vi "CD Init.vi"(0 "Device Reference":T14 format="%.0x", 11 "Error (in)":errorcluster) -> (1 "Card Parameters (out)":T13, 3 "Output Channel Data []":T4[](array[typedef]) {"Labels Settings"."Word"."Param Setting"."Num Bits" min=1 max=32; "Labels Settings"."Word"."Param Setting"."Start Bit" min=8 max=31; "Labels Settings"."Label" format="%.0o"}, 4 "# of Output Channels":i32, 6 "# of Input Channels":i32, 10 "Refs":i32[](array[numeric]), 12 "Map":T3[](array[typedef]), 13 "Raw Values":T1, 14 "Input Channel Data []":T4[](array[typedef]) {"Labels Settings"."Word"."Param Setting"."Num Bits" min=1 max=32; "Labels Settings"."Word"."Param Setting"."Start Bit" min=8 max=31; "Labels Settings"."Label" format="%.0o"}, 15 "Error (out)":errorcluster)   [LabVIEW 2016, in "Ballard Arinc-429 Engine.lvlib"]
uses:
  Ballard Arinc-429 Engine.lvlib
  <vilib>/NI Veristand/Custom Device API/Custom Device Item Ref.ctl
  RT Controls/Card Parameters.ctl
  RT Controls/RT HW Channel.ctl
  RT Controls/RT Label Settings.ctl
  Shared/Controls and Global/Label.ctl
  Shared/Controls and Global/transferPeriod.ctl
  RT Controls/RT Word Settings.ctl
  RT Controls/RT Param Setting.ctl
  Shared/Controls and Global/Start Bit.ctl
  Shared/Controls and Global/Number of Bits.ctl
  Shared/Controls and Global/TransferType.ctl
  RT Controls/RT Tx Association.ctl
  RT Controls/RT Tx Default Raw Value.ctl
  RT Controls/RT Tx Default Raw Value_Association.ctl
  RT Controls/RT Init States.ctl
  <vilib>/NI Veristand/Custom Device API/Custom Device Channel Type.ctl
  <vilib>/NI Veristand/Custom Device Tools/Custom Device Utility Library/RT Debug String Color Spec.ctl
  Shared/Controls and Global/Global.vi
  <vilib>/NI Veristand/Custom Device API/Get Item Property (I32).vi
  <vilib>/NI Veristand/Custom Device API/Get Item Property (Variant).vi
  <vilib>/NI Veristand/Custom Device Tools/Custom Device Utility Library/NI VeriStand - Search for Item by GUID.vi
  <vilib>/NI Veristand/Custom Device API/Custom Device API.lvlib
  Shared/Ballard Arinc-429 Shared.lvlib
  <vilib>/NI Veristand/Custom Device Tools/Custom Device Utility Library/Custom Device Utility Library.lvlib
  <instrlib>/BTI429Lib/BTI429LV.lvlib
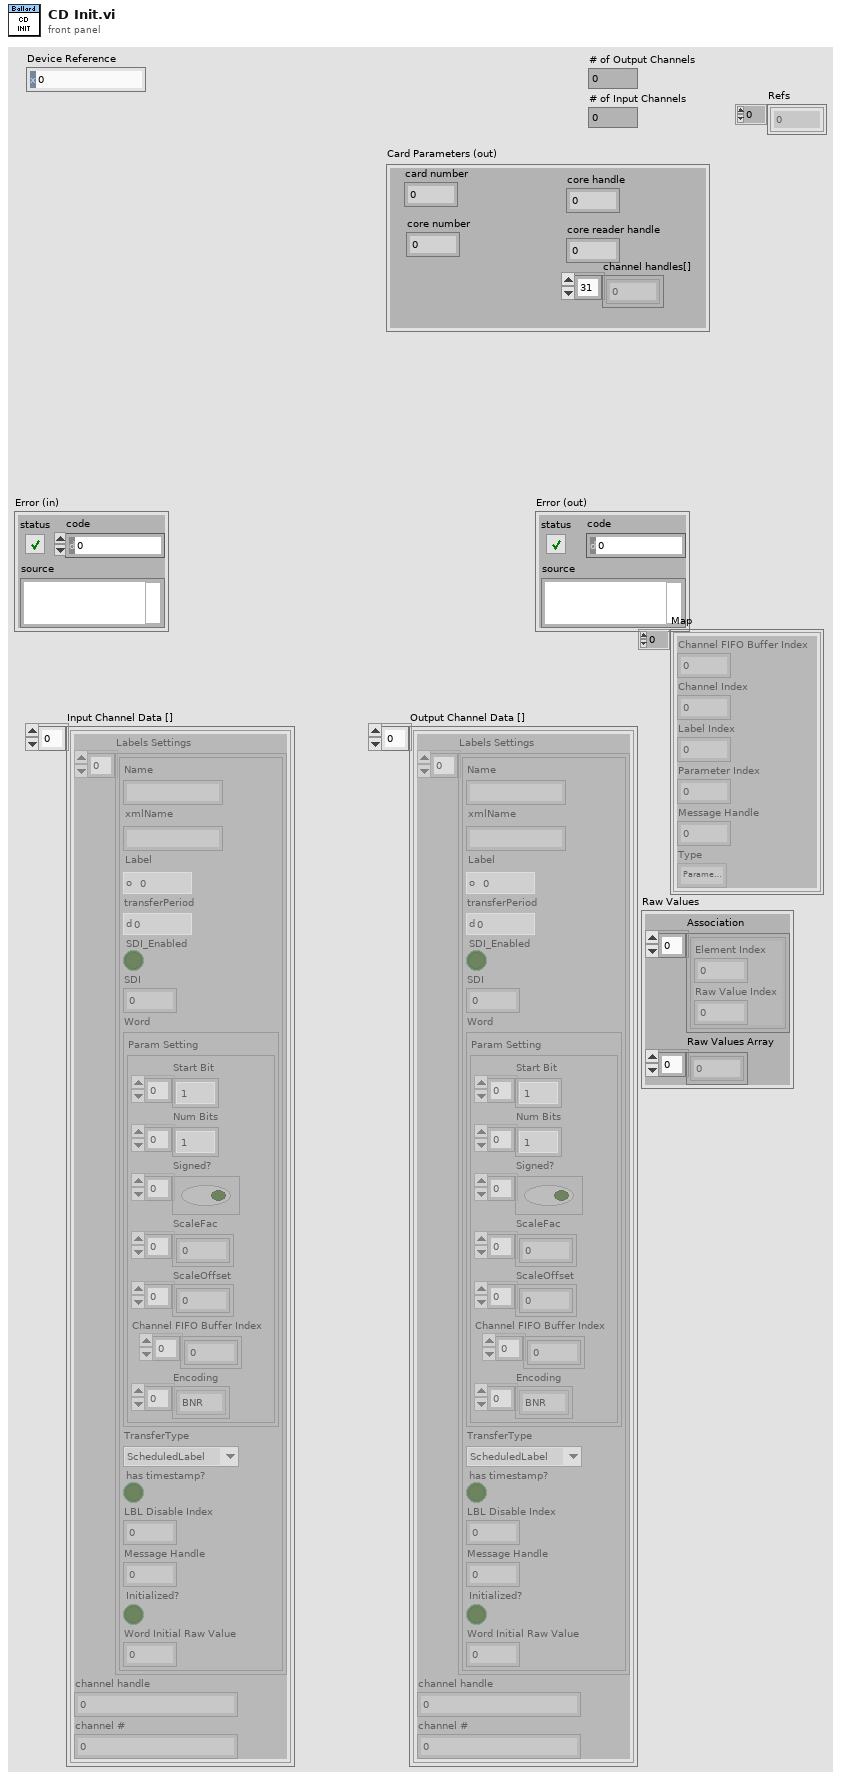
[diagram p1: front panel]
types:
  T1 = typedef "Ballard Arinc-429 Engine.lvlib/RT Tx Default Raw Value.ctl" = cluster{"Association":T2[], "Raw Values Array":u32[]}
  T2 = typedef "Ballard Arinc-429 Engine.lvlib/RT Tx Default Raw Value_Association.ctl" = cluster{"Element Index":i32, "Raw Value Index":i32}
  T3 = typedef "Ballard Arinc-429 Engine.lvlib/RT Tx Association.ctl" = cluster{"Channel FIFO Buffer Index":i32, "Channel Index":i32, "Label Index":i32, "Parameter Index":i32, "Message Handle":u64, "Type":enum16{"Parameter Channel", "Disable Channel"}}
  T4 = typedef "Ballard Arinc-429 Engine.lvlib/RT HW Channel.ctl" = cluster{"Labels Settings":T5[], "channel handle":u32, "channel #":u16}
  T5 = typedef "Ballard Arinc-429 Engine.lvlib/RT Label Settings.ctl" = cluster{"Name":string, "xmlName":string, "Label":T6, "transferPeriod":T7, "SDI_Enabled":bool, "SDI":u8, "Word":T8, "TransferType":T12, "has timestamp?":bool, "LBL Disable Index":i32, "Message Handle":u64, "Initialized?":bool, "Word Initial Raw Value":u32}
  T6 = typedef "Ballard Arinc-429 Shared.lvlib/Label.ctl" = u8
  T7 = typedef "Ballard Arinc-429 Shared.lvlib/transferPeriod.ctl" = u32
  T8 = typedef "Ballard Arinc-429 Engine.lvlib/RT Word Settings.ctl" = cluster{"Param Setting":T9}
  T9 = typedef "Ballard Arinc-429 Engine.lvlib/RT Param Setting.ctl" = cluster{"Start Bit":T10[], "Num Bits":T11[], "Signed?":bool[], "ScaleFac":dbl[], "ScaleOffset":dbl[], "Channel FIFO Buffer Index":i32[], "Encoding":enum16{"BNR", "BCD", "Discrete"}[]}
  T10 = typedef "Ballard Arinc-429 Shared.lvlib/Start Bit.ctl" = i32
  T11 = typedef "Ballard Arinc-429 Shared.lvlib/Number of Bits.ctl" = i32
  T12 = typedef "Ballard Arinc-429 Shared.lvlib/TransferType.ctl" = enum16{"ScheduledLabel", "Acyclic", "Block", "Strobe"}
  T13 = typedef "Ballard Arinc-429 Engine.lvlib/Card Parameters.ctl" = cluster{"card number":i32, "core number":i32, "core handle":u64, "core reader handle":u64, "channel handles[]":u64[]}
  T14 = typedef "Custom Device API.lvlib/Custom Device Item Ref.ctl" = u64
  T15 = typedef "Ballard Arinc-429 Engine.lvlib/RT Init States.ctl" = enum16{"Initialization", "Get Card Settings", "Get Channel Count", "Parse Channels", "Ballard-429 Initialize", "Get Status Channels Reference", "Exit"}
  T16 = typedef "Custom Device API.lvlib/Custom Device Channel Type.ctl" = enum16{"Input", "Output"}
  T17 = enum16{"open", "replace", "create", "open or create", "replace or create", "replace or create with confirmation"}
  T18 = typedef "Custom Device Utility Library.lvlib/RT Debug String Color Spec.ctl" = u16
  T19 = typedef "Custom Device API.lvlib/Custom Device File Dependency.ctl" = cluster{"Source":T20, "RT Destination":path, "ForceDownload?":bool, "SupportedTarget":T22, "Version":string}
  T20 = typedef "Custom Device API.lvlib/Path Specification.ctl" = cluster{"Path":path, "Type":T21}
  T21 = typedef "Custom Device API.lvlib/Path Type.ctl" = enum16{"Absolute", "To Base", "To Common Data Dir", "To Application Data Dir"}
  T22 = typedef "Custom Device API.lvlib/Custom Device Supported Target.ctl" = enum16{"All", "PharLap", "VxWorks", "Windows", "Linux_32_ARM", "Linux_x64", "PharLap & Windows", "PharLap & VxWorks", "VxWorks & Windows"}
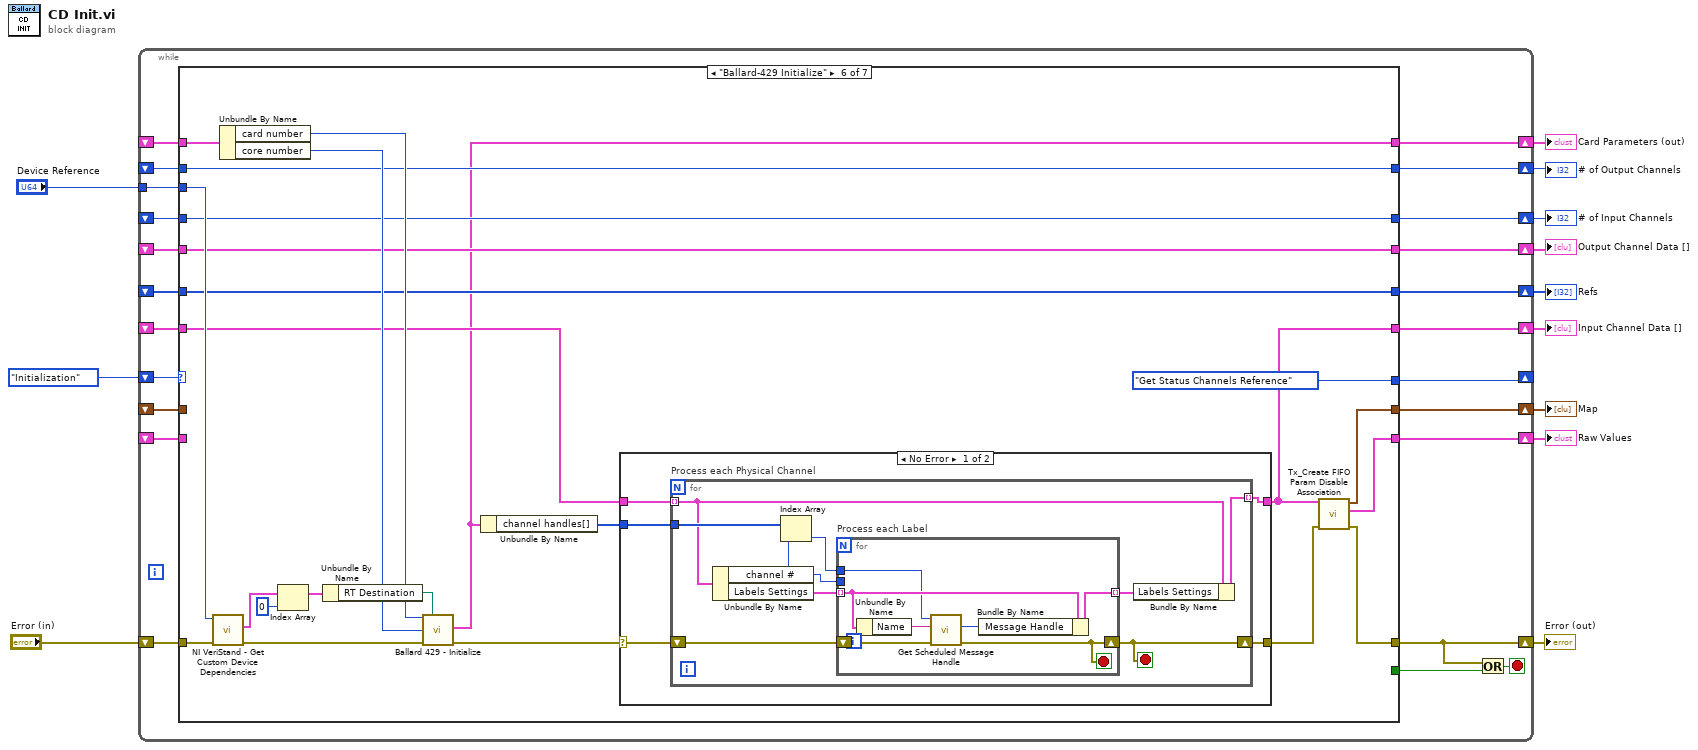
[diagram p0: block diagram]
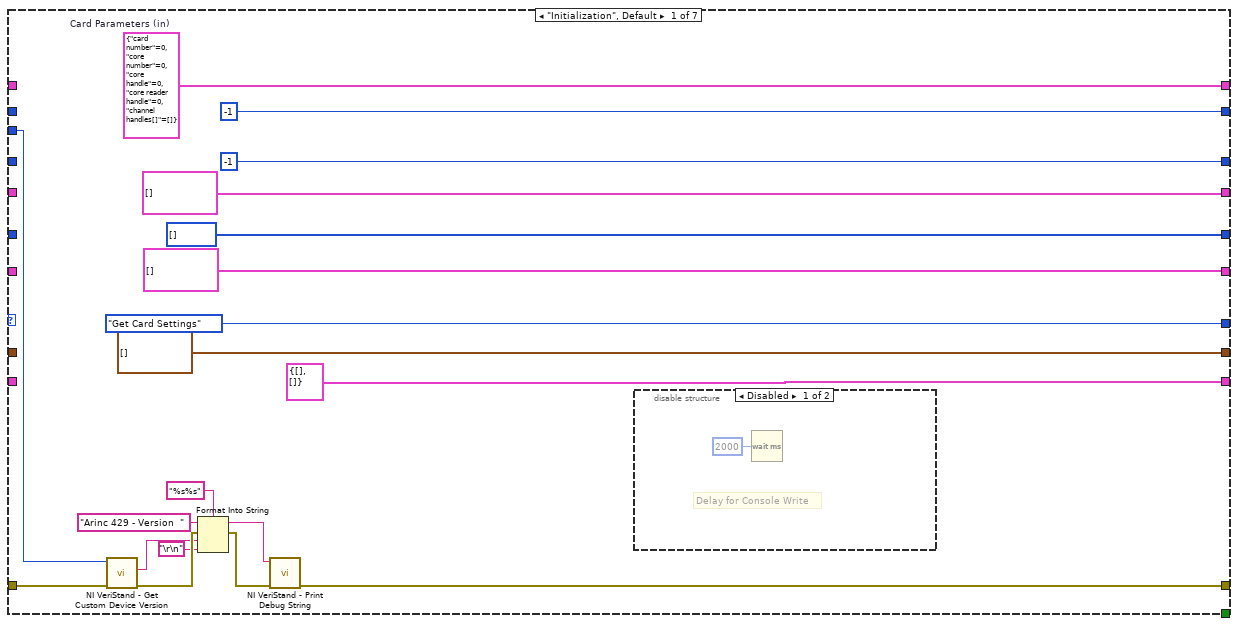
[diagram p2: hidden frame]
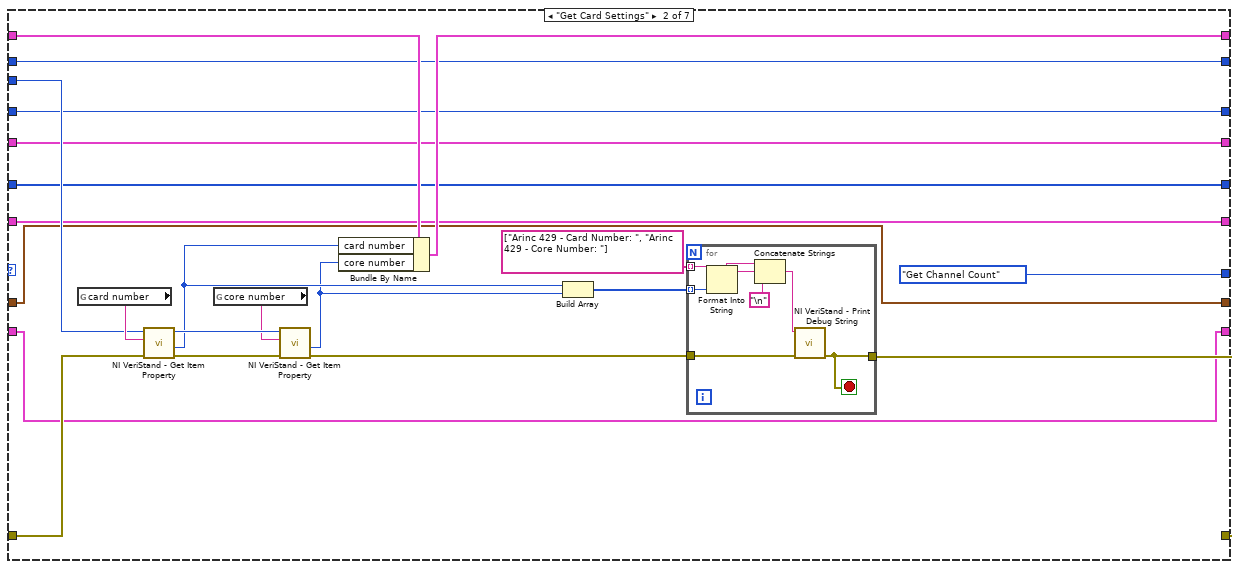
[diagram p4: hidden frame]
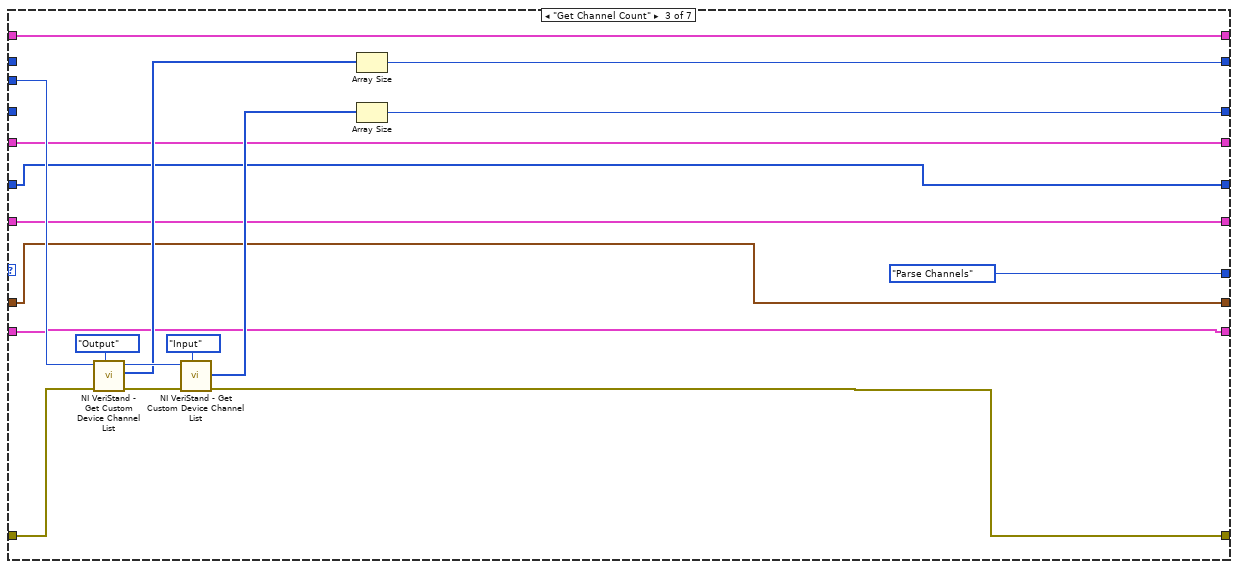
[diagram p5: hidden frame]
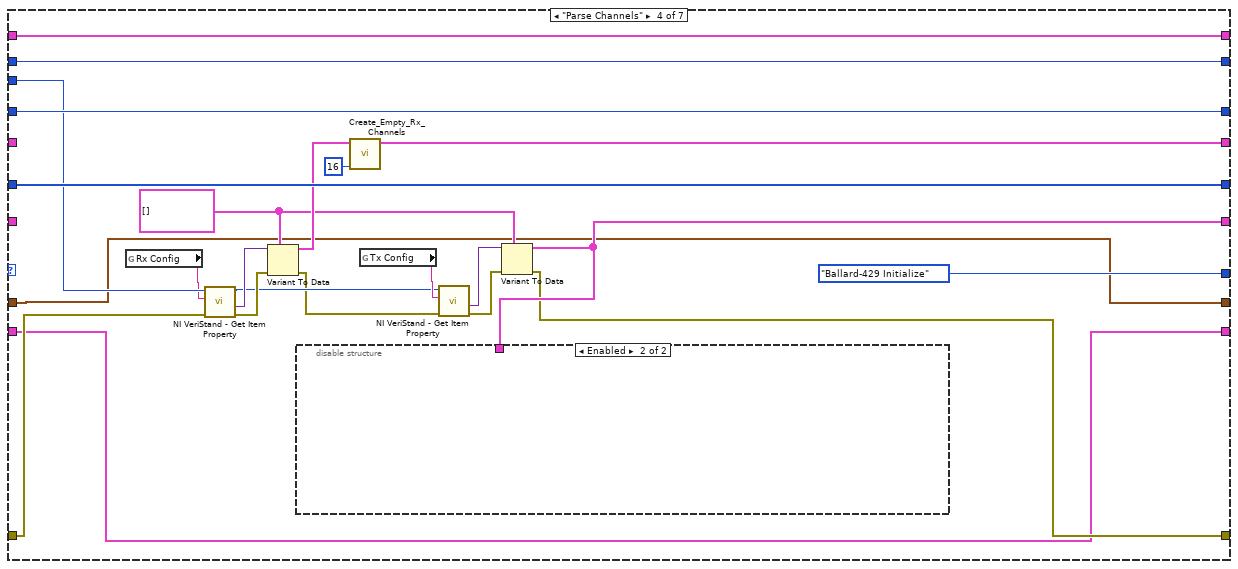
[diagram p6: hidden frame]
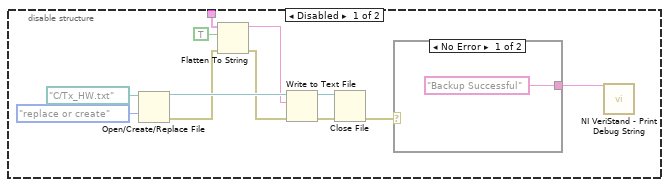
[diagram p7: hidden frame]
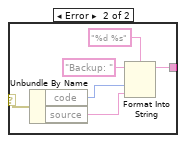
[diagram p8: hidden frame]
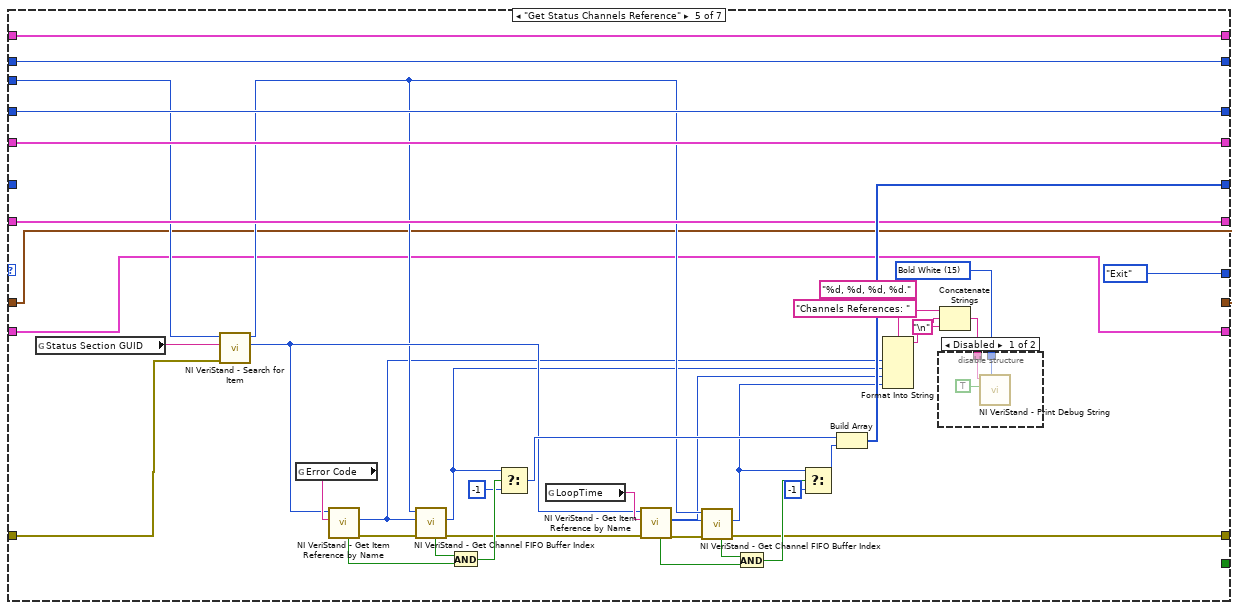
[diagram p9: hidden frame]
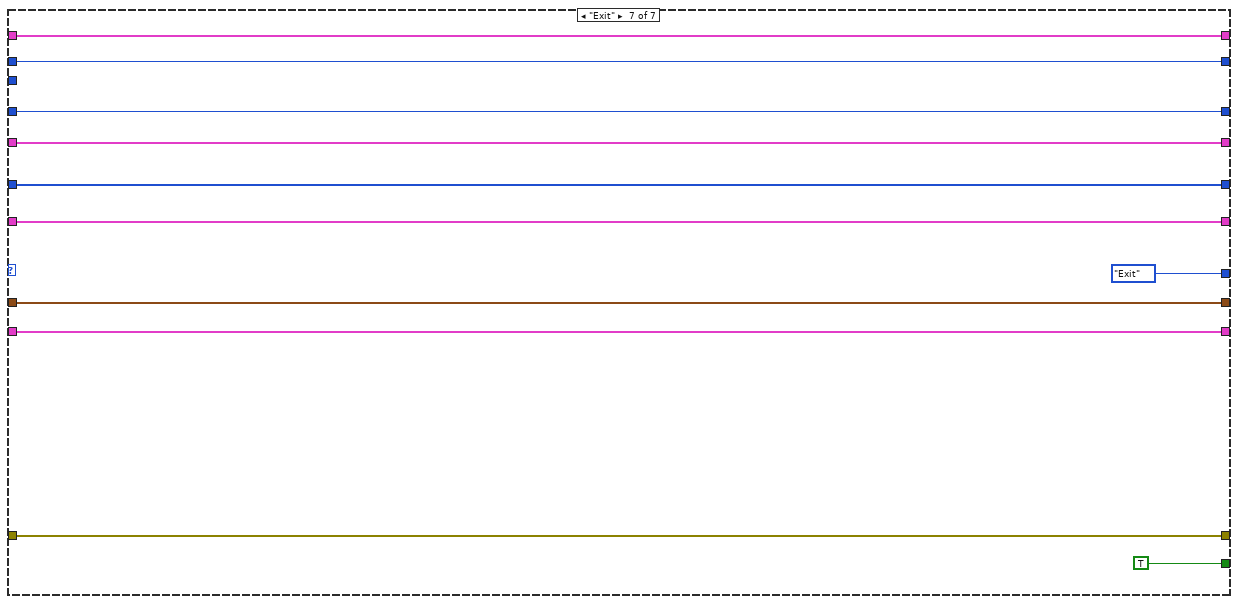
[diagram p12: hidden frame]
diagram:
  n1 = while {
    shift-right: [w34] -> _
    shift-left: RT_Init_States."Initialization" -> [w28]
    tunnel: "Device Reference" -> [w33]
    shift-right: [w29] -> w8
    shift-left: _ -> [w30]
    shift-right: [w27] -> w7
    shift-left: _ -> [w25]
    shift-right: [w26] -> w6
    shift-left: _ -> [w24]
    shift-right: [w23] -> w5
    shift-left: _ -> [w20]
    shift-right: [w22] -> w4
    shift-left: _ -> [w21]
    shift-right: [w19] -> w3
    shift-left: _ -> [w18]
    shift-right: [w17] -> w10
    shift-left: "Error (in)" -> [w35]
    shift-right: [w16] -> w2
    shift-left: _ -> [w15]
    shift-right: [w14] -> w1
    shift-left: _ -> [w13]
    stop <- w32 stop-if-true
    n2 = case shown="\"Ballard-429 Initialize\"" w28 {
      tunnel: w35 -> [w47 w72 w98 w106 w161 w204 w245]
      tunnel: [w45 w69 w85 w105 w162 w188 w245] -> w17
      tunnel: [RT_Init_States."Get Card Settings" RT_Init_States."Get Channel Count" RT_Init_States."Parse Channels" RT_Init_States."Ballard-429 Initialize" RT_Init_States."Exit" RT_Init_States."Get Status Channels Reference" RT_Init_States."Exit"] -> w34
      tunnel: w33 -> [w46 w67 w97 w118 w159 w203 _]
      tunnel: [_ _ _ _ _ _ TRUE] -> w31
      tunnel: w30 -> [_ w66 w93 w124 w174 w208 w242]
      tunnel: [w53 w65 w93 w124 w174 w196 w242] -> w29
      tunnel: [T4[] [] ("Rx Channels Out") w62 w91 w122 w184 w200 w239] -> w27
      tunnel: [T4[] [] ("Channel Data []") w61 w90 w107 w177 w192 w238] -> w26
      tunnel: w25 -> [_ w62 w91 _ w184 w200 w239]
      tunnel: w24 -> [_ w61 w90 _ w177 w201 w238]
      tunnel: [-1 w59 w92 w120 w183 w199 w240] -> w23
      tunnel: [-1 w60 w88 w121 w182 w198 w241] -> w22
      tunnel: w21 -> [_ w60 _ w121 w182 w198 w241]
      tunnel: w20 -> [_ w59 _ w120 w183 w199 w240]
      tunnel: [i32[] [] w58 w89 w119 w178 w197 w237] -> w19
      tunnel: w18 -> [_ w58 w89 w119 _ w197 w237]
      tunnel: [T3[] [] ("Map") w57 w87 w104 w146 w190 w236] -> w16
      tunnel: w15 -> [_ w57 w87 w104 w146 _ w236]
      tunnel: [T1 {"Association"=[], "Raw Values Array"=[]} ("Raw Values") w56 w86 w103 w145 w189 w235] -> w14
      tunnel: w13 -> [_ w56 w86 w103 w145 _ w235]
      frame "Initialization", Default {
        w53 = T13 {"card number"=0, "core number"=0, "core handle"=0, "core reader handle"=0, "channel handles[]"=[]}  # Card Parameters (in)
        n3 = call <vilib>:"NI VeriStand - Get Custom Device Version.vi"("error in (no error)"=w47, "Device Ref in"=w46) -> ("error out"=w44:errorcluster, "Value"=w41:string)  [unwired: 7 in, 1 out]
        n4 = Format Into String(format string="%s%s", initial string="Arinc 429 - Version  ", error in=w44, w41, "\r\n") -> (resulting string=w39:string, error out=w43:errorcluster)
        n5 = call <vilib>:"NI VeriStand - Print Debug String.vi"("error in (no error)"=w43, "Message"=w39) -> ("error out"=w45:errorcluster)  [unwired: 9 in]
        n6 = disable-structure shown="Disabled" {
          frame Disabled {
            # "Delay for Console Write"
            n7 = Wait (ms)(milliseconds to wait=u32 2000) -> ()  [unwired: 1 out]
          }
          frame Enabled {
          }
        }
      }
      frame "Get Card Settings" {
        n8 = global read "Global.vi" "card number"() -> (w73:string)
        n9 = call-poly <vilib>:"NI VeriStand - Get Item Property.vi"("error in (no error)"=w72, "Property Name"=w73, "Item Ref in"=w67) -> ("error out"=w71:errorcluster, "Value"=w64:i32, "Item Ref out"=w75:T14)  [unwired: 5 in, 1 out]
        n10 = global read "Global.vi" "core number"() -> (w74:string)
        n11 = call-poly <vilib>:"NI VeriStand - Get Item Property.vi"("error in (no error)"=w71, "Property Name"=w74, "Item Ref in"=w75) -> ("error out"=w70:errorcluster, "Value"=w63:i32)  [unwired: 5 in, 2 out]
        n12 = Bundle By Name(cluster=w66, "card number"=w64, "core number"=w63) -> (w65:T13)
        n13 = Build Array(w64, w63) -> (w77:i32[])
        n14 = for {
          tunnel: string[] ["Arinc 429 - Card Number: ", "Arinc 429 - Core Number: "] -> [w84] mode=indexing
          tunnel: w77 -> [w83] mode=indexing
          tunnel: w70 -> [w79]
          tunnel: [w78] -> w69
          stop <- w78 stop-if-true
          n15 = Format Into String(w83) -> (resulting string=w82:string)  [unwired: 3 in, 1 out]
          n16 = Concatenate Strings(w84, w82, "\n") -> (w81:string)
          n17 = call <vilib>:"NI VeriStand - Print Debug String.vi"("error in (no error)"=w79, "Message"=w81) -> ("error out"=w78:errorcluster)  [unwired: 9 in]
        }
      }
      frame "Get Channel Count" {
        n18 = call <vilib>:"NI VeriStand - Get Custom Device Channel List.vi"("Channel Type"=Custom_Device_Channel_Type."Output", "error in (no error)"=w98, "Device Ref in"=w97) -> ("error out"=w100:errorcluster, "Specified Channel Ref List"=w96:T14[], "Device Ref out"=w102:T14)  [unwired: 6 out]
        n19 = call <vilib>:"NI VeriStand - Get Custom Device Channel List.vi"("Channel Type"=Custom_Device_Channel_Type."Input", "error in (no error)"=w100, "Device Ref in"=w102) -> ("error out"=w85:errorcluster, "Specified Channel Ref List"=w95:T14[])  [unwired: 7 out]
        n20 = Array Size(array=w96) -> (size(s)=w88:i32)
        n21 = Array Size(array=w95) -> (size(s)=w92:i32)
      }
      frame "Parse Channels" {
        w108 = T4[] [] ("Channel Data []")
        n22 = global read "Global.vi" "Rx Config"() -> (w114:string)
        n23 = call-poly <vilib>:"NI VeriStand - Get Item Property.vi"("error in (no error)"=w106, "Property Name"=w114, "Item Ref in"=w118) -> ("error out"=w117:errorcluster, "Value"=w116:variant, "Item Ref out"=w110:T14)  [unwired: 5 in, 1 out]
        n24 = Variant To Data(error in=w117, type=w108, Variant=w116) -> (data=w115:T4[], error out=w109:errorcluster)
        n25 = call "Create_Empty_Rx_Channels.vi"("Nb Channels"=16, "Rx Channels In"=w115) -> ("Rx Channels Out"=w122:T4[])  [unwired: 9 in]
        n26 = global read "Global.vi" "Tx Config"() -> (w113:string)
        n27 = call-poly <vilib>:"NI VeriStand - Get Item Property.vi"("error in (no error)"=w109, "Property Name"=w113, "Item Ref in"=w110) -> ("error out"=w111:errorcluster, "Value"=w112:variant)  [unwired: 5 in, 2 out]
        n28 = Variant To Data(error in=w111, type=w108, Variant=w112) -> (data=w107:T4[], error out=w105:errorcluster)
        n29 = disable-structure shown="Enabled" {
          disable-tunnel: w107 -> [w136 _]
          frame Disabled {
            n30 = Open/Create/Replace File(file path (use dialog)=path "C:/Tx_HW.txt", operation (0:open)=T17."replace or create") -> (refnum out=w134:refnum<file>, error out=w130:errorcluster)  [unwired: 4 in, 1 out]
            n31 = Flatten To String(anything=w136, prepend array or string size? (T)=TRUE, error in (no error)=w130) -> (data string=w133:string, error out=w129:errorcluster)  [unwired: 1 in, 1 out]
            n32 = Write to Text File(file (use dialog)=w134, text=w133, error in=w129) -> (refnum out=w131:refnum<file>, error out=w132:errorcluster)  [unwired: 1 in, 1 out]
            n33 = Close File(refnum=w131, error in=w132) -> (error out=w128:errorcluster)  [unwired: 1 out]
            n34 = case shown="No Error" w128 {
              selector: w128 -> [_ w143]
              tunnel: ["Backup Successful" ("Message") w144] -> w127
              frame No Error {
              }
              frame Error {
                n35 = Unbundle By Name(w143) -> ("code"=w142:i32, "source"=w141:string)
                n36 = Format Into String(format string="%d %s", initial string="Backup: ", w142, w141) -> (resulting string=w144:string)  [unwired: 1 in, 1 out]
              }
            }
            n37 = call <vilib>:"NI VeriStand - Print Debug String.vi"("Message"=w127) -> ()  [unwired: 10 in, 1 out]
          }
          frame Enabled {
          }
        }
      }
      frame "Get Status Channels Reference" {
        w147 = T18 15 items=["Plain White"=7, "Bold White"=15, "Bold Blue"=9, "Bold Green"=10, "Bold Red"=12] ("Attribute")
        n38 = global read "Global.vi" "Status Section GUID"() -> (w160:string)
        n39 = call-poly <vilib>:"NI VeriStand - Search for Item.vi"("error in"=w161, "Item GUID"=w160, "Section Ref in"=w159) -> ("Item Ref"=w158:T14, "Section Ref out"=w157:T14)  [unwired: 5 in, 2 out]
        n40 = global read "Global.vi" "Error Code"() -> (w176:string)
        n41 = call <vilib>:"NI VeriStand - Get Item Reference by Name.vi"("Item Name"=w176, "Parent Ref in"=w158) -> ("error out"=w173:errorcluster, "Item Ref"=w152:T14, "Found"=w171:bool)  [unwired: 6 in, 1 out]
        n42 = call <vilib>:"NI VeriStand - Get Channel FIFO Buffer Index.vi"("error in"=w173, "Channel Ref"=w152, "Device Ref in"=w157) -> ("error out"=w168:errorcluster, "Channel FIFO Buffer Index"=w151:i32, "Found"=w172:bool)  [unwired: 4 in, 2 out]
        n43 = And(x=w172, y=w171) -> (x .and. y?=w170:bool)
        n44 = Select(t=w151, s=w170, f=-1) -> (s? t:f=w175:i32)
        n45 = global read "Global.vi" "LoopTime"() -> (w180:string)
        n46 = call <vilib>:"NI VeriStand - Get Item Reference by Name.vi"("error in (no error)"=w168, "Item Name"=w180, "Parent Ref in"=w158) -> ("error out"=w166:errorcluster, "Item Ref"=w150:T14, "Found"=w165:bool)  [unwired: 5 in, 1 out]
        n47 = call <vilib>:"NI VeriStand - Get Channel FIFO Buffer Index.vi"("error in"=w166, "Channel Ref"=w150, "Device Ref in"=w157) -> ("error out"=w162:errorcluster, "Channel FIFO Buffer Index"=w149:i32, "Found"=w167:bool)  [unwired: 4 in, 2 out]
        n48 = And(x=w167, y=w165) -> (x .and. y?=w164:bool)
        n49 = Select(t=w149, s=w164, f=-1) -> (s? t:f=w179:i32)
        n50 = Build Array(w175, w179) -> (w178:i32[])
        n51 = Format Into String(format string="%d, %d, %d, %d.", w152, w151, w150, w149) -> (resulting string=w153:string)  [unwired: 2 in, 1 out]
        n52 = Concatenate Strings("Channels References: " ("string"), w153, "\n") -> (w156:string)
        n53 = disable-structure shown="Disabled" {
          disable-tunnel: w156 -> [w187 _]
          disable-tunnel: w147 -> [w186 _]
          frame Disabled {
            n54 = call <vilib>:"NI VeriStand - Print Debug String.vi"("Attribute"=w186, "Add to log file? (T)"=TRUE, "Message"=w187) -> ()  [unwired: 8 in, 1 out]
          }
          frame Enabled {
          }
        }
      }
      frame "Ballard-429 Initialize" {
        n55 = call <vilib>:"NI VeriStand - Get Custom Device Dependencies.vi"("error in (no error)"=w204, "Device Ref in"=w203) -> ("error out"=w193:errorcluster, "Dependencies"=w206:T19[])  [unwired: 7 in, 1 out]
        n56 = Unbundle By Name(w208) -> ("card number"=w210:i32, "core number"=w209:i32)
        n57 = Index Array(array=w206, index=0) -> (element=w205:T19)
        n58 = Unbundle By Name(w205) -> ("RT Destination"=w202:path)
        n59 = call "Ballard 429 - Initialize.vi"("Card Number"=w210, "RT Config Filepath"=w202, "Core Number"=w209, "Error (in)"=w193) -> ("Card Parameters (out)"=w196:T13, "Error (out)"=w194:errorcluster)  [unwired: 10 in]
        n60 = Unbundle By Name(w196) -> ("channel handles[]"=w207:u64[])
        n61 = case shown="No Error" w194 {
          selector: w194 -> [w212 w233]
          tunnel: w207 -> [w216 _]
          tunnel: w201 -> [w215 w234]
          tunnel: [w214 w234] -> w192
          tunnel: [w213 w233] -> w191
          frame No Error {
            n62 = for "Process each Physical Channel" {
              tunnel: w215 -> [w221] mode=indexing
              tunnel: w216 -> [w225]
              tunnel: [w220] -> w214 mode=indexing
              shift-right: [w217] -> w213
              shift-left: w212 -> [w223]
              stop <- w217 stop-if-true
              n63 = Unbundle By Name(w221) -> ("channel #"=w218:u16, "Labels Settings"=w222:T5[])
              n64 = Index Array(array=w225, index=w218) -> (element=w224:u64)
              n65 = for "Process each Label" {
                tunnel: w222 -> [w231] mode=indexing
                tunnel: w224 -> [w227]
                tunnel: [w230] -> w219 mode=indexing
                shift-right: [w226] -> w217
                shift-left: w223 -> [w232]
                tunnel: w218 -> [_]
                stop <- w226 stop-if-true
                n66 = Unbundle By Name(w231) -> ("Name"=w229:string)
                n67 = call <instrlib>:"Get Scheduled Message Handle.vi"("error in (no error)"=w232, "message name"=w229, "channel handle in"=w227) -> ("error out"=w226:errorcluster, "message handle out"=w228:u64)  [unwired: 6 in, 1 out]
                n68 = Bundle By Name(cluster=w231, "Message Handle"=w228) -> (w230:T5)
              }
              n69 = Bundle By Name(cluster=w221, "Labels Settings"=w219) -> (w220:T4)
            }
          }
          frame Error {
          }
        }
        n70 = call "Tx_Create FIFO Param Disable Association.vi"("error in (no error)"=w191, "Input Channel Data []"=w192) -> ("error out"=w188:errorcluster, "Raw Values"=w189:T1, "Map"=w190:T3[])  [unwired: 7 in]
      }
      frame "Exit" {
      }
    }
    n71 = Or(x=w17, y=w31) -> (x .or. y?=w32:bool)
  }
  "Error (out)" <- w10
  "Card Parameters (out)" <- w8
  "Output Channel Data []" <- w7
  "Input Channel Data []" <- w6
  "# of Output Channels" <- w4
  "# of Input Channels" <- w5
  "Refs" <- w3
  "Map" <- w2
  "Raw Values" <- w1
